vi "OptimalAngel.vi"(11 "Joystick X":dbl) -> (3 "Angel":dbl)   [LabVIEW 2011]
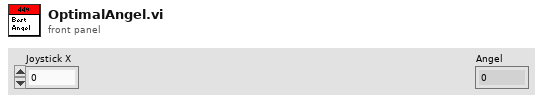
[diagram p1: front panel]
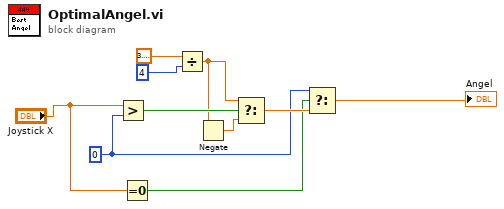
[diagram p0: block diagram]
diagram:
  w2 = 0
  n1 = Greater?(x="Joystick X", y=w2) -> (0:w10:bool)
  n2 = Equal To 0?(x="Joystick X") -> (x = 0?=w5:bool)
  n3 = Divide(x=3.141592653589793, y=4) -> (x/y=w3:dbl)
  n4 = Negate(x=w3) -> (-x=w4:dbl)
  n5 = Select(t=w3, s=w10, f=w4) -> (s? t:f=w6:dbl)
  n6 = Select(t=w2, s=w5, f=w6) -> (s? t:f=→"Angel":dbl)
